vi "GDX_ACC_GyroPosition.vi"(8 "dt":dbl, 9 "Y Gyro (rad/s)":dbl, 10 "X Gyro (rad/s)":dbl, 11 "Initialize":bool) -> (0 "GyroX Roll":dbl, 1 "GyroX Radians (Roll)":dbl, 2 "GyroY Pitch":dbl, 3 "GyroY Radians (Pitch)":dbl)   [LabVIEW 2019]
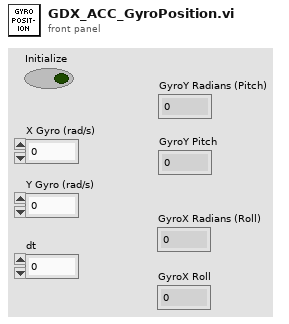
[diagram p1: front panel]
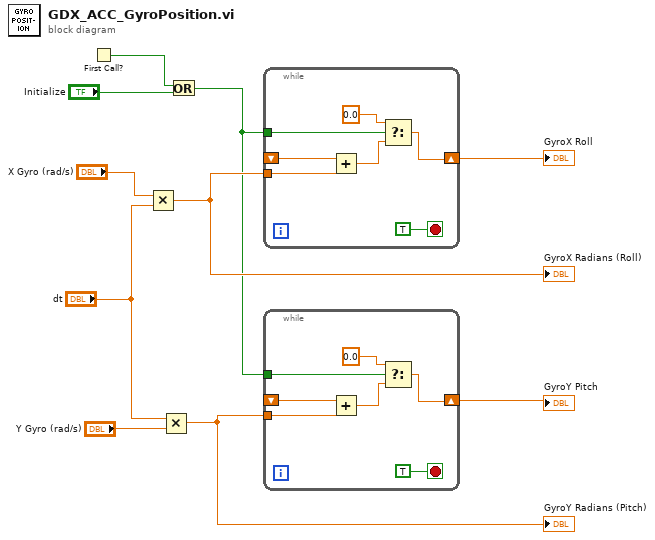
[diagram p0: block diagram]
diagram:
  n1 = First Call?() -> (First Call?: T/F=w9:bool)
  n2 = Multiply(x="X Gyro (rad/s)", y="dt") -> (x*y=w6:dbl)
  "GyroX Radians (Roll)" <- w6
  n3 = Multiply(x="dt", y="Y Gyro (rad/s)") -> (x*y=w2:dbl)
  "GyroY Radians (Pitch)" <- w2
  n4 = Or(x=w9, y="Initialize") -> (x .or. y?=w3:bool)
  n5 = while {
    tunnel: w6 -> [w11]
    shift-right: [w13] -> w10
    shift-left: _ -> [w17]
    tunnel: w3 -> [w15]
    stop <- TRUE stop-if-true
    n6 = Add(x=w17, y=w11) -> (x+y=w14:dbl)
    n7 = Select(t=0.0, s=w15, f=w14) -> (s? t:f=w13:dbl)
  }
  "GyroX Roll" <- w10
  n8 = while {
    tunnel: w2 -> [w18]
    shift-right: [w20] -> w1
    shift-left: _ -> [w24]
    tunnel: w3 -> [w22]
    stop <- TRUE stop-if-true
    n9 = Add(x=w24, y=w18) -> (x+y=w21:dbl)
    n10 = Select(t=0.0, s=w22, f=w21) -> (s? t:f=w20:dbl)
  }
  "GyroY Pitch" <- w1
